vi "moving_average.vi"(1 "Input":dbl) -> (0 "Output":dbl)   [LabVIEW 2011]
doc: "Moving average,\n\nThis program calculates and displays the moving average, with a pre-selected number. First of all, the program initialized two shift registers. The top shift register is initialized with one element and this register continiously adds the previous value with the new value. This shift register keeps the total of the last xx measurements. When dividing the results of the add function with the pre-selected value, we can calculate the moving average value. The bottom shift register contains an array with the dimension \"Average\". This shift register keeps all values of the measurement. The replacement function replaces every loop the new value. \n \nThis method is very efficent and fast, because we using the replace element function inside the loop and before we enter the while loop we initialzes the array. This VI was created in LabVIEW 6.1."
panel:
  in  "stop":bool
  out "?":cluster{dbl, dbl}(graph)
  in  "Average":i32=25
  # "Select the moving average and then\nrun the VI.  The chart will show the\ncurrent measurement and the \nresulting moving average."
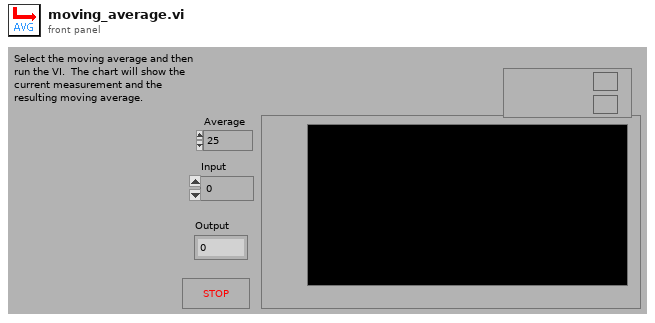
[diagram p1: front panel]
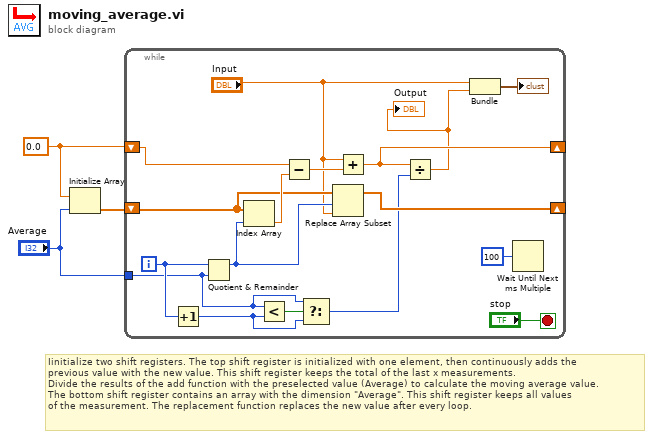
[diagram p0: block diagram]
diagram:
  w1 = 0.0 ("y")
  # "Iinitialize two shift registers. The top shift register is initialized with one element, then continuously adds the \nprevious value with the new value. This shift register keeps the total of the last x measurements. \nDivide the results of the add function with the preselected value (Average) to calculate the moving average value.\nThe bottom shift register contains an array with the dimension \"Average\". This shift register keeps all values \nof the measurement. The replacement function replaces the new value after every loop."
  n1 = Initialize Array(w1, "Average") -> (w3:dbl[])
  n2 = while {
    tunnel: "Average" -> [w6]
    shift-left: w3 -> [w18]
    shift-right: [w20] -> _
    shift-left: w1 -> [w16]
    shift-right: [w14] -> _
    i -> [w11]
    stop <- "stop" stop-if-true
    n3 = Increment(x=w11) -> (x+1=w8:i32)
    n4 = Quotient & Remainder(x=w11, y=w6) -> (x-y*floor(x/y)=w15:i32)  [unwired: 1 out]
    n5 = Index Array(array=w18, index=w15) -> (element=w19:dbl)
    n6 = Less?(x=w6, y=w8) -> (x < y?=w10:bool)
    n7 = Subtract(x=w16, y=w19) -> (x-y=w17:dbl)
    n8 = Select(t=w6, s=w10, f=w8) -> (s? t:f=w9:i32)
    n9 = Replace Array Subset(array=w18, new element="Input", index=w15) -> (w20:dbl[])
    n10 = Add(x="Input", y=w17) -> (x+y=w14:dbl)
    n11 = Divide(x=w14, y=w9) -> (x/y=w4:dbl)
    "Output" <- w4
    n12 = Bundle("Input"="Input", w4) -> (→"?":cluster{"Input":dbl, dbl})  [unwired: 1 in]
    n13 = Wait Until Next ms Multiple(millisecond multiple=u32 100) -> ()  [unwired: 1 out]
  }
